vi "time_conversion.vi"(11 "array_time":u8[](array[numeric])) -> (3 "time_U64":u64)   [LabVIEW 2018]
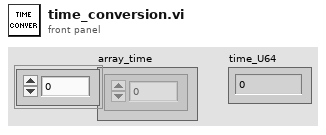
[diagram p1: front panel]
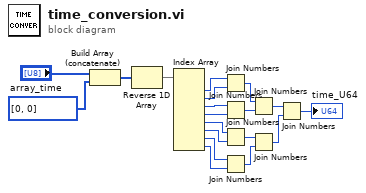
[diagram p0: block diagram]
diagram:
  n1 = Build Array (concatenate)("array_time", u8[] [0, 0] ("element")) -> (w18:u8[])
  n2 = Reverse 1D Array(array=w18) -> (reversed array=w19:u8[])
  n3 = Index Array(array=w19) -> (element #1=w3:u8, element #2=w4:u8, element #3=w5:u8, element #4=w6:u8, element #5=w7:u8, element #6=w8:u8, element #7=w9:u8, element #8=w10:u8)  [unwired: 8 in]
  n4 = Join Numbers(hi=w3, lo=w4) -> ((hi.lo)=w12:u16)
  n5 = Join Numbers(hi=w5, lo=w6) -> ((hi.lo)=w11:u16)
  n6 = Join Numbers(hi=w7, lo=w8) -> ((hi.lo)=w14:u16)
  n7 = Join Numbers(hi=w9, lo=w10) -> ((hi.lo)=w13:u16)
  n8 = Join Numbers(hi=w12, lo=w11) -> ((hi.lo)=w16:u32)
  n9 = Join Numbers(hi=w14, lo=w13) -> ((hi.lo)=w15:u32)
  n10 = Join Numbers(hi=w16, lo=w15) -> ((hi.lo)=→"time_U64":u64)
